vi "Task_03_sub_01.vi"(11 "Array":u8[](array[numeric])) -> (2 "Stat_Cluster":T2, 3 "Histogram Graph":T1)   [LabVIEW 2018]
doc: "Этот ВПП вычислияет максимум, минимум, RMS и Mean для массива чисел, а также строит для выборки гистограму распределения."
uses:
  <vilib>/Analysis/baseanly.llb/Mean (DBL).vi
  <vilib>/Analysis/5stat.llb/RMS (DBL).vi
  <vilib>/Analysis/NI_AALBase.lvlib
  <vilib>/Analysis/NI_AALPro.lvlib
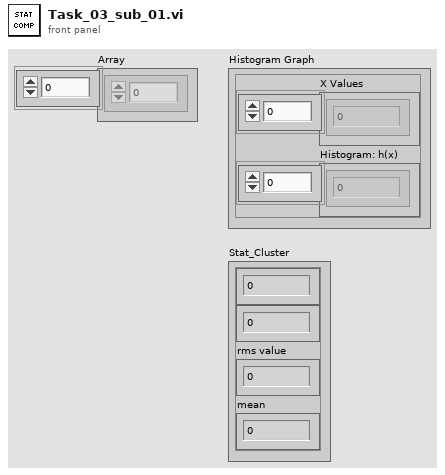
[diagram p1: front panel]
types:
  T1 = cluster{"X Values":dbl[], "Histogram: h(x)":i32[]}
  T2 = cluster{"Numeric Control":u8, "Numeric Control":u8, "rms value":dbl, "mean":dbl}
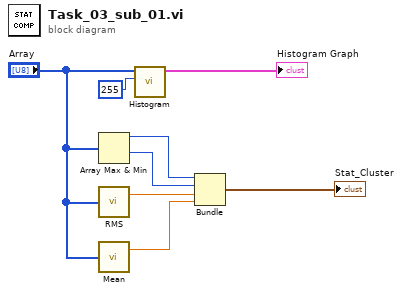
[diagram p0: block diagram]
diagram:
  n1 = Array Max & Min(array="Array") -> (max value=w4:u8, min value=w5:u8)  [unwired: 2 out]
  n2 = call-poly <vilib>:"RMS.vi"("X"="Array") -> ("rms value"=w6:dbl)  [unwired: 1 out]
  n3 = call-poly <vilib>:"Mean.vi"("X"="Array") -> ("mean"=w7:dbl)  [unwired: 1 out]
  n4 = call <vilib>:"Histogram.vi"("intervals"=255, "X"="Array") -> ("Histogram Graph"=→"Histogram Graph":T1)  [unwired: 6 in, 3 out]
  n5 = Bundle(w4, w5, "rms value"=w6, "mean"=w7) -> (→"Stat_Cluster":cluster{u8, u8, "rms value":dbl, "mean":dbl})  [unwired: 1 in]
